vi "Write ACK Packet.vi"(8 "error in":errorcluster, 11 "ELAN data unit (ADU) in":refnum<class "ELAN Data Unit.lvclass">) -> (0 "error out":errorcluster, 3 "ELAN data unit (ADU) out":refnum<class "ELAN Data Unit.lvclass">)   [LabVIEW 2021, in "ELAN Data Unit.lvclass"]
uses:
  ELAN Data Unit.lvclass
  ELAN Data Unit.lvclass/ELAN Data Unit.ctl
  <vilib>/Utility/error.llb/Error Cluster From Error Code.vi
  <vilib>/ErrorRing/Error Ring.xnode
  Modbus_v121c/Network Interface/Serial Interface/Serial Shared Components/Serial Shared Components.lvlib
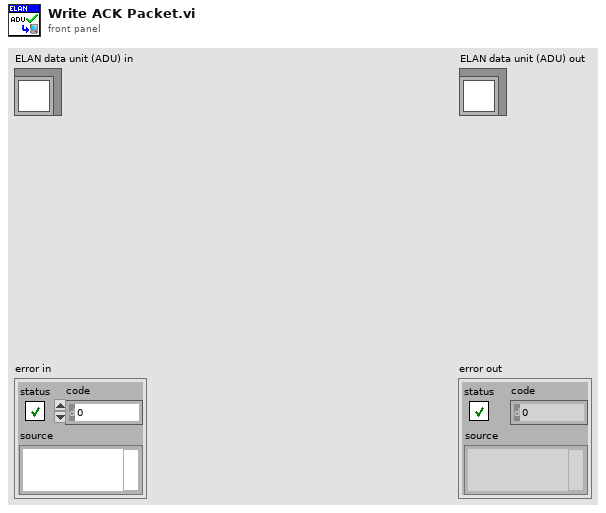
[diagram p1: front panel]
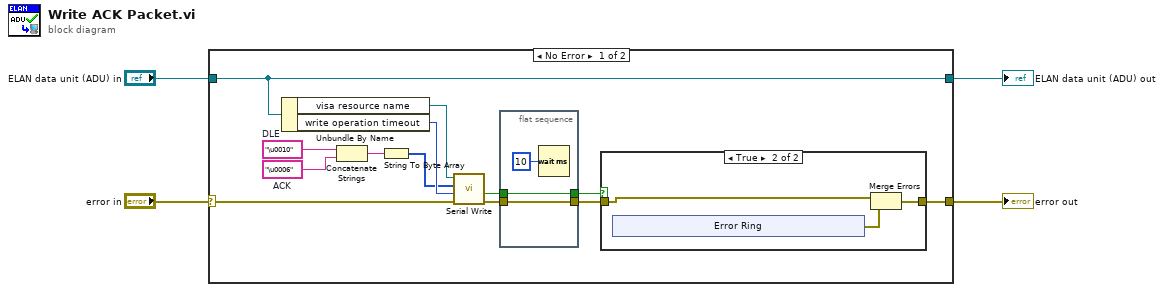
[diagram p0: block diagram]
diagram:
  n1 = case shown="No Error" "error in" {
    selector: "error in" -> [w9 w30]
    tunnel: [w17 w30] -> w2
    tunnel: "ELAN data unit (ADU) in" -> [w11 w29]
    tunnel: [w11 w29] -> w3
    frame No Error {
      w16 = "\u0006"  # ACK
      w15 = "\u0010"  # DLE
      n2 = Unbundle By Name(w11) -> ("visa resource name"=w13:refnum<visa-resource-name>, "write operation timeout"=w12:u32)
      n3 = Concatenate Strings(w15, w16) -> (w14:string)
      n4 = String To Byte Array(string=w14) -> (unsigned byte array=w10:u8[])
      n5 = call "Serial Write.vi"("error in"=w9, "timeout (ms)"=w12, "data"=w10, "Visa Resource"=w13) -> ("error out"=w7:errorcluster, "timed out?"=w8:bool)  [unwired: 6 in]
      n6 = flat-sequence {
        tunnel: w8 -> [w18]
        tunnel: w7 -> [w19]
        tunnel: [w19] -> w6
        tunnel: [w18] -> w5
        frame #0 {
          n7 = Wait (ms)(milliseconds to wait=u32 10 ("millisecond multiple")) -> ()  [unwired: 1 out]
        }
      }
      n8 = case shown="True" w5 {
        tunnel: w6 -> [w21 w23]
        tunnel: [w21 w24] -> w17
        frame False {
        }
        frame True {
          n9 = xnode "Error Ring"() -> ("error out"=w22:errorcluster)
          n10 = Merge Errors(w23, w22) -> (w24:errorcluster)
        }
      }
    }
    frame Error {
    }
  }
  "error out" <- w2
  "ELAN data unit (ADU) out" <- w3
